vi "testwin32event.vi"() -> ()   [LabVIEW 2011]
uses:
  kernel32.dll
panel:
  out "HANDLE CreateEvent":u32
  out "数值输入控件":i32
  in  "布尔":bool
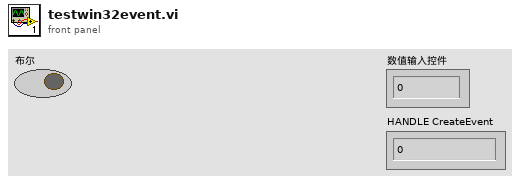
[diagram p1: front panel]
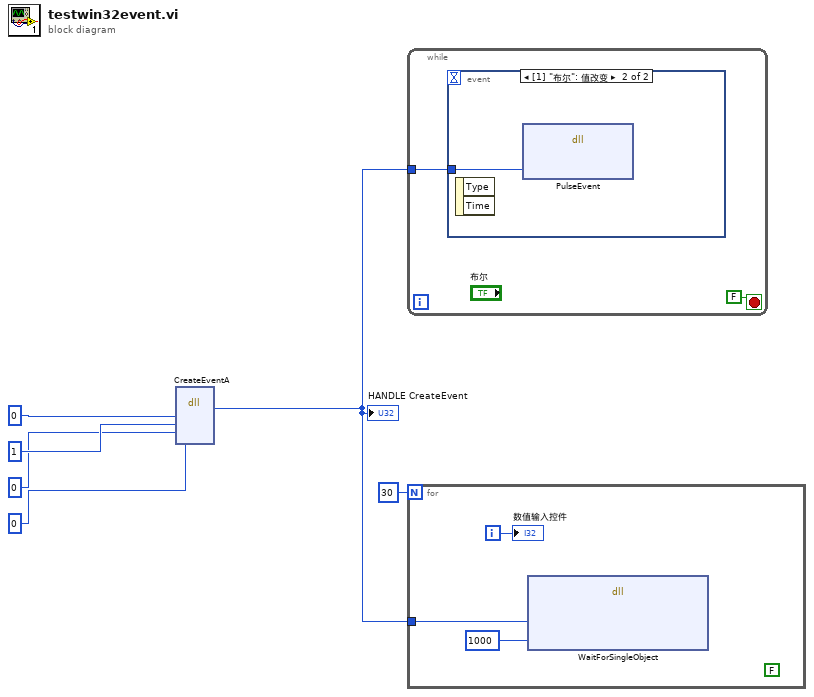
[diagram p0: block diagram]
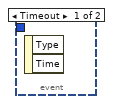
[diagram p2: hidden frame]
diagram:
  n1 = dll-call lib="kernel32.dll" fn="CreateEventA"("LPSECURITY_ATTRIBUTES lpEventAttributes"=i8 0, "BOOL bManualReset"=i8 1, "BOOL bInitialState"=i8 0, "LPCTSTR lpName"=i8 0) -> ("HANDLE CreateEvent"=w3:i32)  [unwired: 7 in, 2 out]
  "HANDLE CreateEvent" <- w3
  n2 = while {
    tunnel: w3 -> [w7]
    stop <- FALSE stop-if-true
    n3 = event shown="[1] \"布尔\": 值改变" {
      selector: _ -> [_ _]
      dyn-events: _ -> [_ _]
      timeout: _ -> [_ _]
      tunnel: w7 -> [_ w9]
      event Timeout {
        n4 = event-data() -> ()  [unwired: 1 in, 2 out]
      }
      event "布尔": Value Change {
        n5 = event-data() -> ()  [unwired: 1 in, 2 out]
        n6 = dll-call lib="kernel32.dll" fn="PulseEvent"("HANDLE"=w9) -> ()  [unwired: 5 in, 2 out]
      }
    }
  }
  n7 = for {
    N: 30 -> [_]
    tunnel: w3 -> [w12]
    i -> [w10]
    (unwired) FALSE
    n8 = dll-call lib="kernel32.dll" fn="WaitForSingleObject"("HANDLE hHandle"=w12, "DWORD dwMilliseconds"=u32 1000) -> ()  [unwired: 6 in, 2 out]
    "数值输入控件" <- w10
  }
